vi "increment-tool-count.vi"(10 "tool# or drive subsystem name":string, 11 "Tool array in":T1[](array[typedef])) -> (3 "Tool array out":T1[](array[typedef]))   [LabVIEW 2017, in "labview-standard-library.lvlib" / "automode-scripting.lvlib"]
uses:
  automode-scripting.lvlib
  type-defs/tool-call-tracker.ctl
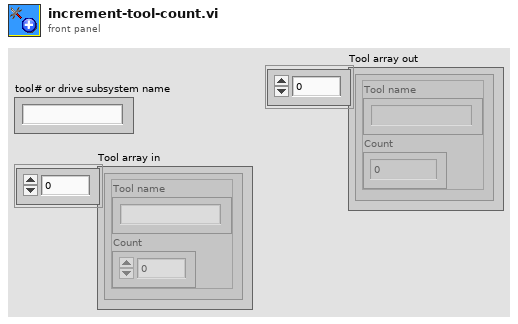
[diagram p1: front panel]
types:
  T1 = typedef "tool-call-tracker.ctl" = cluster{"Tool name":string, "Count":i32}
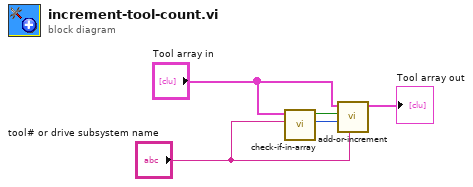
[diagram p0: block diagram]
diagram:
  n1 = call "check-if-in-array.vi"("tool# or drive subsystem name"="tool# or drive subsystem name", "Tool array in"="Tool array in") -> ("Position if found"=w2:i32, "Found?"=w5:bool)  [unwired: 8 in]
  n2 = call "add-or-increment.vi"("tool# or drive subsystem name"="tool# or drive subsystem name", "Position if found"=w2, "Found?"=w5, "Tool array in"="Tool array in") -> ("Tool array out"=→"Tool array out":T1[])  [unwired: 7 in]
